vi "Hot_Wire_Setup.vi"(1 "XW?":bool, 2 "Setup String":string) -> (0 "Output string":string="\rBridge 1\tNewcastle Bridge\rProbe type\t\rWire ID\t\rOverheat ratio 1\t0.500000\rGain 1\t0.000000\rLP Filter Hz 1\t0.000000\r")   [LabVIEW 2010]
uses:
  Controls/Metal_Type.ctl
  Controls/ok_button.ctl
  Globals/Constants_global.vi
panel:
  in  "Wire ID number":string
  in  "Probe type":u16(ring) items=["P01 (Straight, plated)", "P05 (Boundary, plated)", "P11 (Straight, miniature)", "P12 (Slant, miniature)", "P14 (Bent, miniature)", "P31 (Thermo)", "P51(Dual slant, plated)", "P51/120 (Dual slant, plated)", "P53(BL Dual slant, plated)", "P61 (Dual slant, min)", "P62 (Dual Cross, Min)", "P64 (Cross bent Min)", "P76 (Straight, temp. comp.)", "R61 (Dual Parallel, film)"]
  in  "Edit Probe Types":bool
  in  "Edit Bridge Types":bool
  in  "Ok":T1
  in  "Instrument setup":T3(array[cluster])=[{"Gain"=0.0, "LP Filter Hz"=0, "Bridge"=4, "Overheat ratio"=0.5, "Wire"="", "Offset Voltage"=0.0, "Metal Type"=enum."Tungsten"}] {"Offset Voltage" min=0.0 max=10.0 format="%#.2f"; "Overheat ratio" min=0.5 max=0.99 format="%.2f"; "Bridge" items=["DISA 56 C14", "DISA 56 C16", "DISA 56 C17", "Newcastle Bridge", "PSI 6110"]; "Gain" min=1.0 max=100.0 format="%.2f"}
  # "Rhot-Rcold\n   Rcold"
  # "V=Gain(E-Offset)"
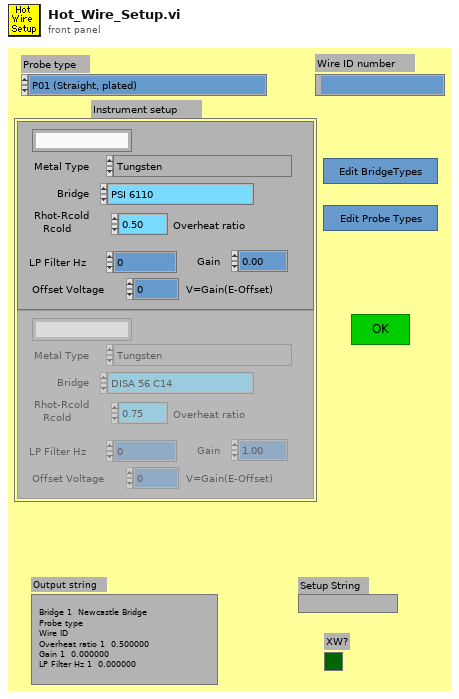
[diagram p1: front panel]
types:
  T1 = typedef "ok_button.ctl" = bool
  T2 = typedef "Metal_Type.ctl" = enum16{"Tungsten", "Platinum", "Platinum-plated Tungsten"}
  T3 = cluster{"Gain":dbl, "LP Filter Hz":i32, "Bridge":u16, "Overheat ratio":dbl, "Wire":string, "Offset Voltage":dbl, "Metal Type":T2}[]
  T4 = cluster{"Gain":dbl, "LP Filter Hz":i32, "Bridge":u16, "Overheat ratio":dbl, "Wire":string, "Offset Voltage":dbl, "Metal Type":T2}
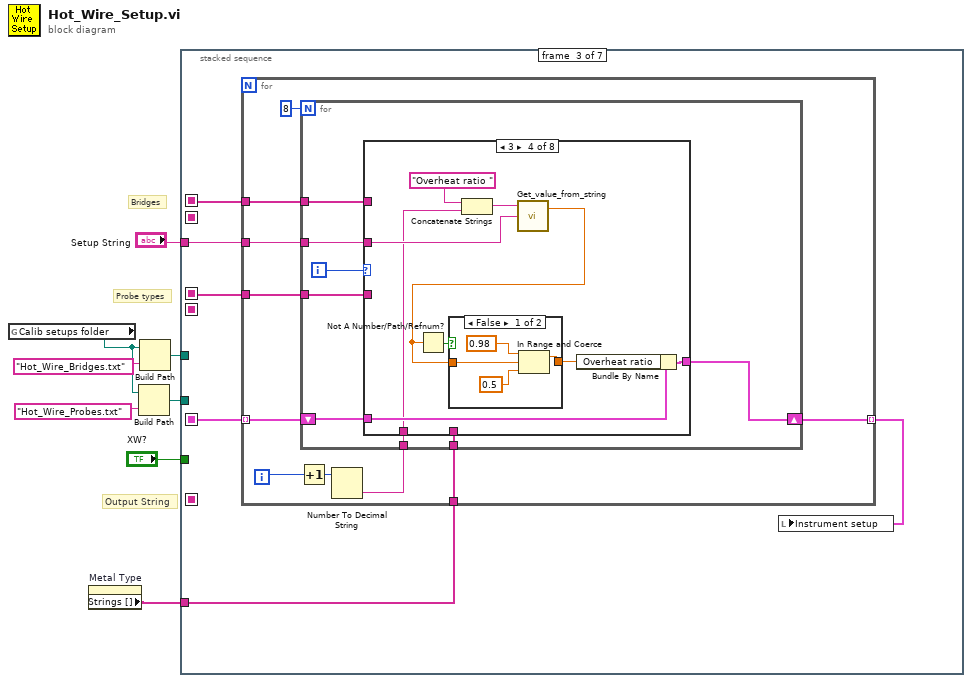
[diagram p0: block diagram]
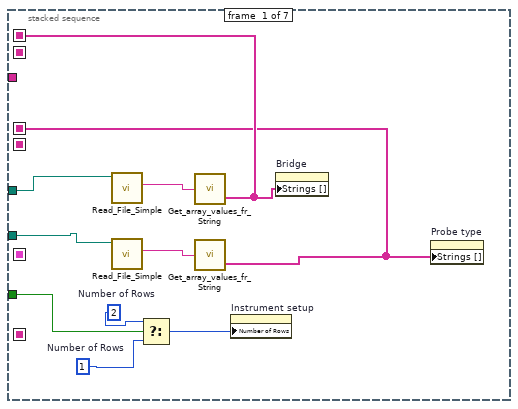
[diagram p2: hidden frame]
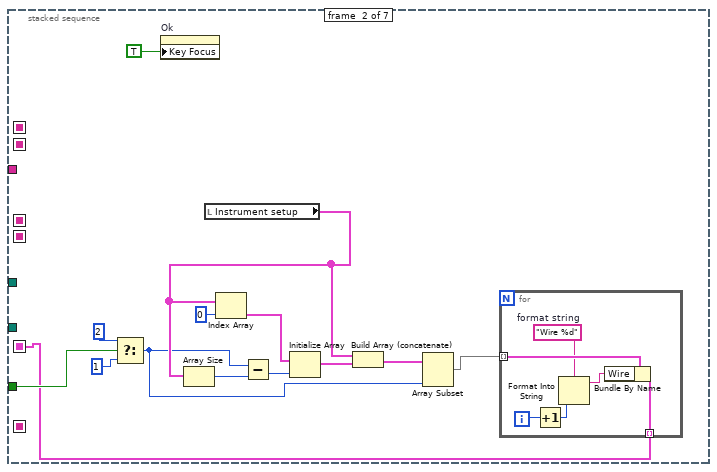
[diagram p3: hidden frame]
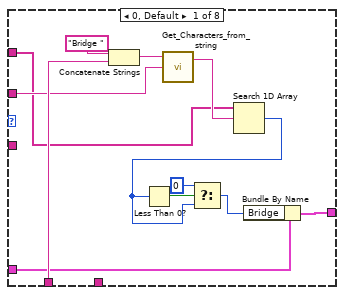
[diagram p4: hidden frame]
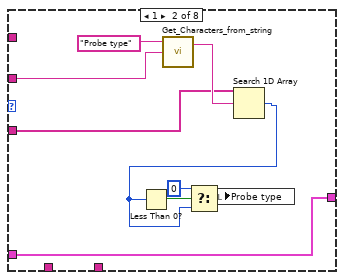
[diagram p5: hidden frame]
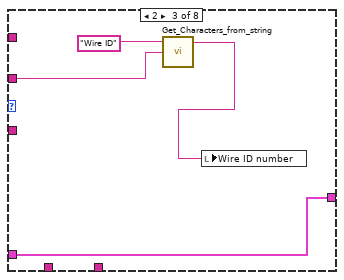
[diagram p6: hidden frame]
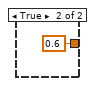
[diagram p7: hidden frame]
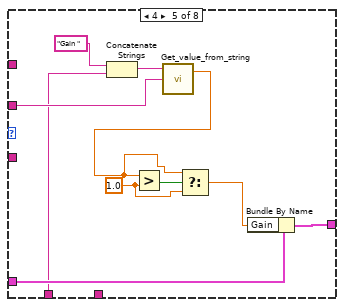
[diagram p8: hidden frame]
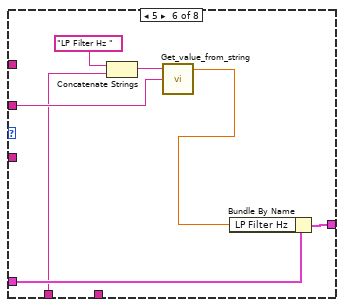
[diagram p9: hidden frame]
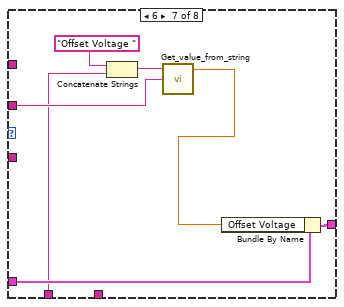
[diagram p10: hidden frame]
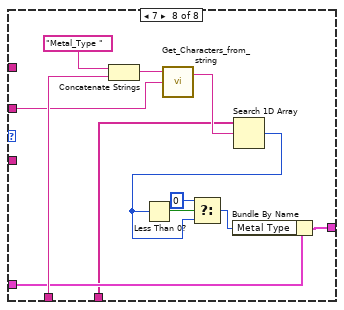
[diagram p11: hidden frame]
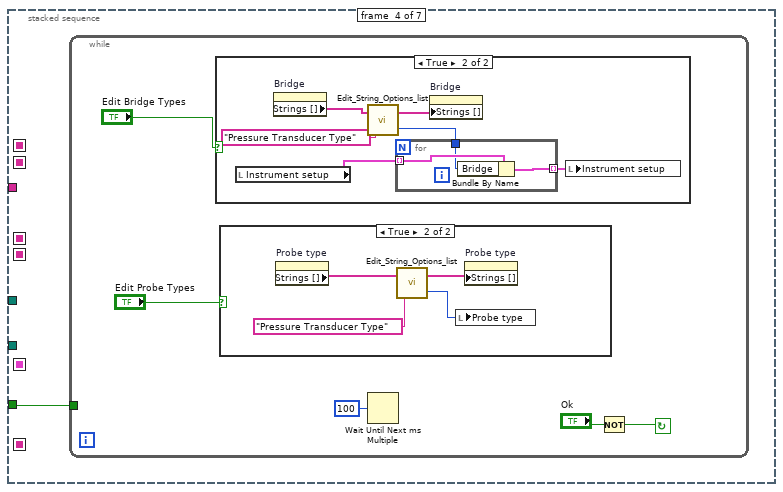
[diagram p12: hidden frame]
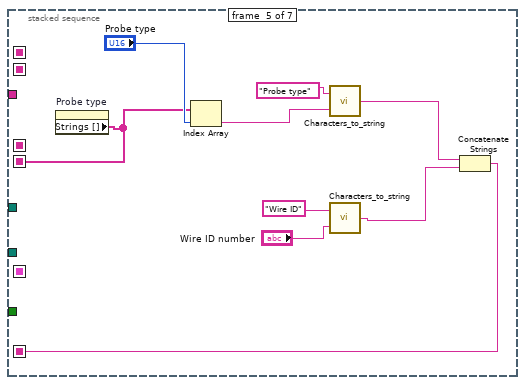
[diagram p15: hidden frame]
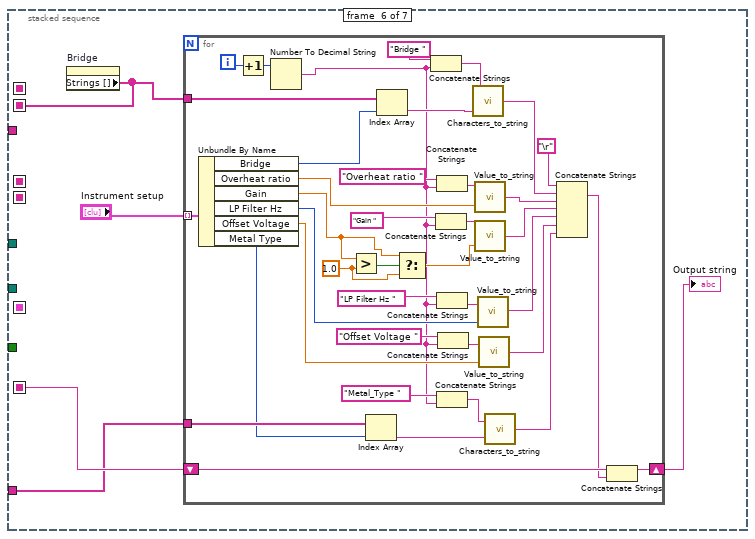
[diagram p16: hidden frame]
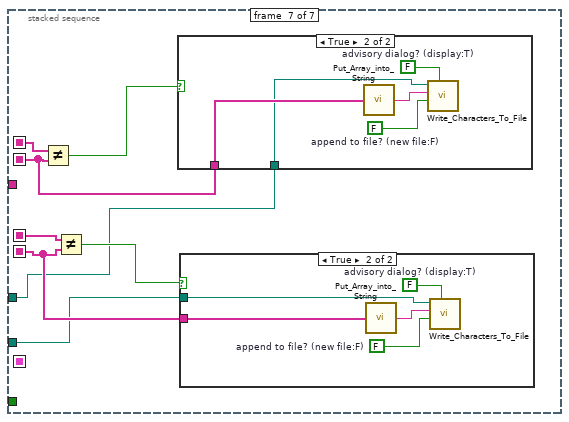
[diagram p17: hidden frame]
diagram:
  # "Probe types"
  # "Bridges"
  # "Output String"
  n1 = global read "Constants_global.vi" "Calib setups folder"() -> (w3:path)
  n2 = property on="Metal Type" class="Enum (strict)"() -> ("Strings []"=w1:string[])  [unwired: 2 in, 2 out]
  n3 = Build Path(base path=w3, name or relative path="Hot_Wire_Probes.txt") -> (appended path=w2:path)
  n4 = Build Path(base path=w3, name or relative path="Hot_Wire_Bridges.txt") -> (appended path=w5:path)
  n5 = stacked-sequence {
    seq-local: [_ w20 _ _ _ _ _] -> [_ _ w44 _ _ _ _]
    seq-local: [_ _ _ _ w157 _ _] -> [_ _ _ _ _ w169 _]
    seq-local: [w16 _ _ _ _ _ _] -> [_ _ w40 _ _ _ w217]
    seq-local: [w13 _ _ _ _ _ _] -> [_ _ w41 _ _ _ w214]
    seq-local: [_ _ _ _ _ w170 _] -> [_ _ _ _ _ _ w215]
    seq-local: [_ _ _ _ w162 _ _] -> [_ _ _ _ _ _ w213]
    tunnel: "XW?" -> [w12 w26 _ w138 _ _ _]
    tunnel: "Setup String" -> [_ _ w42 _ _ _ _]
    tunnel: w5 -> [w17 _ _ _ _ _ w210]
    tunnel: w2 -> [w14 _ _ _ _ _ w211]
    tunnel: w1 -> [_ _ w39 _ _ w166 _]
    frame #0 {
      w9 = u32 1  # Number of Rows
      w10 = u32 2  # Number of Rows
      n6 = call "Read_File_Simple.vi"("Filename"=w17) -> ("string"=w18:string)  [unwired: 2 in, 7 out]
      n7 = call "Read_File_Simple.vi"("Filename"=w14) -> ("string"=w15:string)  [unwired: 2 in, 7 out]
      n8 = Select(t=w10, s=w12, f=w9) -> (s? t:f=w11:u32)
      n9 = call "Get_array_values_fr_String.vi"("String Value"=w18) -> ("String array"=w16:string[])  [unwired: 1 out]
      n10 = call "Get_array_values_fr_String.vi"("String Value"=w15) -> ("String array"=w13:string[])  [unwired: 1 out]
      n11 = property on="Instrument setup" class="Arr (strict)"("Number of Rows"=w11) -> ()  [unwired: 2 in, 2 out]
      n12 = property on="Bridge" class="Ring (strict)"("Strings []"=w16) -> ()  [unwired: 2 in, 2 out]
      n13 = property on="Probe type" class="Ring (strict)"("Strings []"=w13) -> ()  [unwired: 2 in, 2 out]
    }
    frame #1 {
      n14 = Select(t=2, s=w26, f=1) -> (s? t:f=w22:i32)
      n15 = property on="Ok" class="Bool"("Key Focus"=TRUE) -> ()  [unwired: 2 in, 2 out]
      n16 = local read "Instrument setup"() -> (w27:T3)
      n17 = Array Size(array=w27) -> (size(s)=w32:i32)
      n18 = Index Array(array=w27, index=0 ("Index")) -> (element=w29:T4)
      n19 = Subtract(x=w22, y=w32) -> (x-y=w31:i32)
      n20 = Initialize Array(w29, w31) -> (w28:T3)
      n21 = Build Array (concatenate)(w27, w28) -> (w23:T3)
      n22 = Array Subset(array=w23, length=w22) -> (w19:T3)  [unwired: 1 in]
      n23 = for {
        tunnel: [w38] -> w20 mode=indexing
        tunnel: w19 -> [w37] mode=indexing
        i -> [w36]
        w34 = "Wire %d"  # format string
        n24 = Increment(x=w36) -> (x+1=w35:i32)
        n25 = Format Into String(format string=w34, w35) -> (resulting string=w33:string)  [unwired: 2 in, 1 out]
        n26 = Bundle By Name(cluster=w37, "Wire"=w33) -> (w38:T4)
      }
    }
    frame #2 {
      n27 = for {
        tunnel: w44 -> [w53] mode=indexing
        tunnel: [w52] -> w43 mode=indexing
        tunnel: w42 -> [w48]
        tunnel: w40 -> [w47]
        tunnel: w41 -> [w46]
        tunnel: w39 -> [w45]
        i -> [w50]
        n28 = Increment(x=w50) -> (x+1=w51:i32)
        n29 = Number To Decimal String(number=w51) -> (decimal integer string=w49:string)  [unwired: 1 out]
        n30 = for {
          N: 8 -> [_]
          shift-right: [w58] -> w52
          shift-left: w53 -> [w61]
          tunnel: w49 -> [w60]
          tunnel: w48 -> [w59]
          tunnel: w47 -> [w57]
          tunnel: w46 -> [w56]
          tunnel: w45 -> [w55]
          i -> [w62]
          n31 = case shown="3" w62 {
            tunnel: w61 -> [w70 w76 w85 w95 w110 w117 w124 w133]
            tunnel: w60 -> [w73 _ _ w92 w107 w113 w120 w136]
            tunnel: w59 -> [w71 w83 w87 w96 w111 w118 w125 w134]
            tunnel: [w68 w76 w85 w94 w109 w116 w123 w131] -> w58
            tunnel: w57 -> [w67 _ _ _ _ _ _ _]
            tunnel: w56 -> [_ w80 _ _ _ _ _ _]
            tunnel: w55 -> [_ _ _ _ _ _ _ w126]
            frame 0, Default {
              n32 = Concatenate Strings("Bridge ", w73) -> (w72:string)
              n33 = call "Get_Characters_from_string.vi"("Input string"=w71, "Variable name"=w72) -> ("Value"=w69:string)  [unwired: 1 in, 1 out]
              n34 = Search 1D Array(1D array=w67, element=w69) -> (index of element=w64:i32)  [unwired: 1 out]
              n35 = Less Than 0?(x=w64) -> (x < 0?=w65:bool)
              n36 = Select(t=0, s=w65, f=w64) -> (s? t:f=w63:i32)
              n37 = Bundle By Name(cluster=w70, "Bridge"=w63) -> (w68:T4)
            }
            frame 1 {
              n38 = call "Get_Characters_from_string.vi"("Input string"=w83, "Variable name"="Probe type") -> ("Value"=w82:string)  [unwired: 1 in, 1 out]
              n39 = Search 1D Array(1D array=w80, element=w82) -> (index of element=w77:i32)  [unwired: 1 out]
              n40 = Less Than 0?(x=w77) -> (x < 0?=w78:bool)
              n41 = Select(t=0, s=w78, f=w77) -> (s? t:f=w75:i32)
              n42 = local write "Probe type"(w75) -> ()
            }
            frame 2 {
              n43 = call "Get_Characters_from_string.vi"("Input string"=w87, "Variable name"="Wire ID") -> ("Value"=w84:string)  [unwired: 1 in, 1 out]
              n44 = local write "Wire ID number"(w84) -> ()
            }
            frame 3 {
              n45 = Concatenate Strings("Overheat ratio ", w92) -> (w91:string)
              n46 = call "Get_value_from_string.vi"("Input string"=w96, "Variable name"=w91) -> ("Value"=w89:dbl)  [unwired: 1 in, 1 out]
              n47 = Not A Number/Path/Refnum?(number/path/refnum=w89) -> (NaN/Path/Refnum?=w88:bool)
              n48 = case shown="False" w88 {
                tunnel: [w98 0.6 ("upper limit")] -> w90
                tunnel: w89 -> [w97 _]
                frame False {
                  n49 = In Range and Coerce(upper limit=0.98, x=w97, lower limit=0.5) -> (coerced(x)=w98:dbl)  [unwired: 1 out]
                }
                frame True {
                }
              }
              n50 = Bundle By Name(cluster=w95, "Overheat ratio"=w90) -> (w94:T4)
            }
            frame 4 {
              w103 = 1.0 ("y")
              n51 = Concatenate Strings("Gain ", w107) -> (w106:string)
              n52 = call "Get_value_from_string.vi"("Input string"=w111, "Variable name"=w106) -> ("Value"=w104:dbl)  [unwired: 1 in, 1 out]
              n53 = Greater?(x=w104, y=w103) -> (0:w105:bool)
              n54 = Select(t=w104, s=w105, f=w103) -> (s? t:f=w102:dbl)
              n55 = Bundle By Name(cluster=w110, "Gain"=w102) -> (w109:T4)
            }
            frame 5 {
              n56 = Concatenate Strings("LP Filter Hz ", w113) -> (w112:string)
              n57 = call "Get_value_from_string.vi"("Input string"=w118, "Variable name"=w112) -> ("Value"=w115:dbl)  [unwired: 1 in, 1 out]
              n58 = Bundle By Name(cluster=w117, "LP Filter Hz"=w115) -> (w116:T4)
            }
            frame 6 {
              n59 = Concatenate Strings("Offset Voltage ", w120) -> (w119:string)
              n60 = call "Get_value_from_string.vi"("Input string"=w125, "Variable name"=w119) -> ("Value"=w122:dbl)  [unwired: 1 in, 1 out]
              n61 = Bundle By Name(cluster=w124, "Offset Voltage"=w122) -> (w123:T4)
            }
            frame 7 {
              n62 = Concatenate Strings("Metal_Type ", w136) -> (w135:string)
              n63 = call "Get_Characters_from_string.vi"("Input string"=w134, "Variable name"=w135) -> ("Value"=w132:string)  [unwired: 1 in, 1 out]
              n64 = Search 1D Array(1D array=w126, element=w132) -> (index of element=w128:i32)  [unwired: 1 out]
              n65 = Less Than 0?(x=w128) -> (x < 0?=w129:bool)
              n66 = Select(t=0, s=w129, f=w128) -> (s? t:f=w127:i32)
              n67 = Bundle By Name(cluster=w133, "Metal Type"=w127) -> (w131:T4)
            }
          }
        }
      }
      n68 = local write "Instrument setup"(w43) -> ()
    }
    frame #3 {
      n69 = while {
        tunnel: w138 -> [_]
        stop <- w143 continue-if-true
        n70 = case shown="True" "Edit Bridge Types" {
          frame False {
          }
          frame True {
            n71 = local read "Instrument setup"() -> (w150:T3)
            n72 = property on="Bridge" class="Ring (strict)"() -> ("Strings []"=w152:string[])  [unwired: 2 in, 2 out]
            n73 = call "Edit_String_Options_list.vi"("Channel Name"="Pressure Transducer Type", "String array"=w152) -> ("New Selection Index"=w148:i32, "String array Out"=w151:string[])
            n74 = for {
              tunnel: w150 -> [w156] mode=indexing
              tunnel: [w155] -> w149 mode=indexing
              tunnel: w148 -> [w154]
              n75 = Bundle By Name(cluster=w156, "Bridge"=w154) -> (w155:T4)
            }
            n76 = property on="Bridge" class="Ring (strict)"("Strings []"=w151) -> ()  [unwired: 2 in, 2 out]
            n77 = local write "Instrument setup"(w149) -> ()
          }
        }
        n78 = case shown="True" "Edit Probe Types" {
          frame False {
          }
          frame True {
            n79 = property on="Probe type" class="Ring (strict)"() -> ("Strings []"=w145:string[])  [unwired: 2 in, 2 out]
            n80 = call "Edit_String_Options_list.vi"("Channel Name"="Pressure Transducer Type", "String array"=w145) -> ("New Selection Index"=w144:i32, "String array Out"=w146:string[])
            n81 = local write "Probe type"(w144) -> ()
            n82 = property on="Probe type" class="Ring (strict)"("Strings []"=w146) -> ()  [unwired: 2 in, 2 out]
          }
        }
        n83 = Wait Until Next ms Multiple(millisecond multiple=u32 100) -> ()  [unwired: 1 out]
        n84 = Not(x="Ok") -> (.not. x?=w143:T1)
      }
    }
    frame #4 {
      n85 = property on="Probe type" class="Ring (strict)"() -> ("Strings []"=w162:string[])  [unwired: 2 in, 2 out]
      n86 = Index Array(array=w162, index="Probe type") -> (element=w161:string)
      n87 = call "Characters_to_string.vi"("Characters to write"=w161, "Label for characters"="Probe type") -> ("Output string"=w158:string)
      n88 = call "Characters_to_string.vi"("Characters to write"="Wire ID number", "Label for characters"="Wire ID") -> ("Output string"=w159:string)
      n89 = Concatenate Strings(w158, w159) -> (w157:string)
    }
    frame #5 {
      n90 = property on="Bridge" class="Ring (strict)"() -> ("Strings []"=w170:string[])  [unwired: 2 in, 2 out]
      n91 = for {
        shift-right: [w203] -> w168
        shift-left: w169 -> [w202]
        tunnel: "Instrument setup" -> [w190] mode=indexing
        tunnel: w170 -> [w189]
        tunnel: w166 -> [w175]
        i -> [w200]
        w180 = 1.0 ("y")
        n92 = Unbundle By Name(w190) -> ("Bridge"=w188:u16, "Overheat ratio"=w204:dbl, "Gain"=w179:dbl, "LP Filter Hz"=w208:i32, "Offset Voltage"=w184:dbl, "Metal Type"=w174:T2)
        n93 = Increment(x=w200) -> (x+1=w199:i32)
        n94 = Number To Decimal String(number=w199) -> (decimal integer string=w176:string)  [unwired: 1 out]
        n95 = Greater?(x=w179, y=w180) -> (0:w181:bool)
        n96 = Index Array(array=w175, index=w174) -> (element=w172:string)
        n97 = Index Array(array=w189, index=w188) -> (element=w205:string)
        n98 = Select(t=w179, s=w181, f=w180) -> (s? t:f=w178:dbl)
        n99 = Concatenate Strings("Bridge ", w176) -> (w197:string)
        n100 = Concatenate Strings("Gain ", w176) -> (w192:string)
        n101 = Concatenate Strings("Overheat ratio ", w176) -> (w195:string)
        n102 = Concatenate Strings("LP Filter Hz ", w176) -> (w191:string)
        n103 = Concatenate Strings("Metal_Type ", w176) -> (w173:string)
        n104 = Concatenate Strings("Offset Voltage ", w176) -> (w185:string)
        n105 = call "Characters_to_string.vi"("Characters to write"=w205, "Label for characters"=w197) -> ("Output string"=w187:string)
        n106 = call "Value_to_string.vi"("Value"=w204, "Label for value"=w195) -> ("Output string"=w206:string)  [unwired: 1 in]
        n107 = call "Value_to_string.vi"("Value"=w178, "Label for value"=w192) -> ("Output string"=w207:string)  [unwired: 1 in]
        n108 = call "Value_to_string.vi"("Value"=w208, "Label for value"=w191) -> ("Output string"=w209:string)  [unwired: 1 in]
        n109 = call "Value_to_string.vi"("Value"=w184, "Label for value"=w185) -> ("Output string"=w182:string)  [unwired: 1 in]
        n110 = call "Characters_to_string.vi"("Characters to write"=w172, "Label for characters"=w173) -> ("Output string"=w171:string)
        n111 = Concatenate Strings("\r", w187, w206, w207, w209, w182, w171) -> (w201:string)
        n112 = Concatenate Strings(w202, w201) -> (w203:string)
      }
      "Output string" <- w168
    }
    frame #6 {
      n113 = Not Equal?(x=w217, y=w215) -> (x != y?=w216:bool)
      n114 = Not Equal?(x=w214, y=w213) -> (x != y?=w212:bool)
      n115 = case shown="True" w216 {
        tunnel: w215 -> [_ w224]
        tunnel: w210 -> [_ w223]
        frame False {
        }
        frame True {
          w225 = FALSE  # append to file? (new file:F)
          w226 = FALSE  # advisory dialog? (display:T)
          n116 = call "Put_Array_into_String.vi"("String array"=w224) -> ("String Value"=w227:string)
          n117 = call "Write_Characters_To_File.vi"("file path (dialog if empty)"=w223, "advisory dialog? (display:T)"=w226, "character string"=w227, "append to file? (new file:F)"=w225) -> ()  [unwired: 1 in, 4 out]
        }
      }
      n118 = case shown="True" w212 {
        tunnel: w213 -> [_ w219]
        tunnel: w211 -> [_ w218]
        frame False {
        }
        frame True {
          w220 = FALSE  # append to file? (new file:F)
          w221 = FALSE  # advisory dialog? (display:T)
          n119 = call "Put_Array_into_String.vi"("String array"=w219) -> ("String Value"=w222:string)
          n120 = call "Write_Characters_To_File.vi"("file path (dialog if empty)"=w218, "advisory dialog? (display:T)"=w221, "character string"=w222, "append to file? (new file:F)"=w220) -> ()  [unwired: 1 in, 4 out]
        }
      }
    }
  }
